vi "Initialize Session without Resources.vi"(11 "error in (no error)":errorcluster) -> (4 "session out":refnum<k21>, 15 "error out":errorcluster)   [LabVIEW 2020, in "SLSC.lvlib"]
doc: "Initializes an SLSC session without specifying any resources or opening any network connections. Use Initialize Session without Resources if you need to set session properties that control network timeouts or the ability to programmatically abort blocking network operations."
uses:
  <vilib>/SLSC/SLSC.lvlib
  nislsclvapi.dll
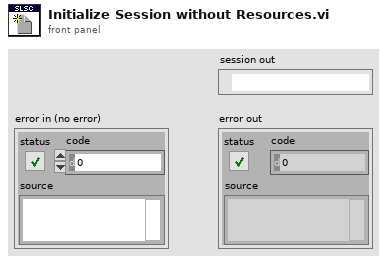
[diagram p1: front panel]
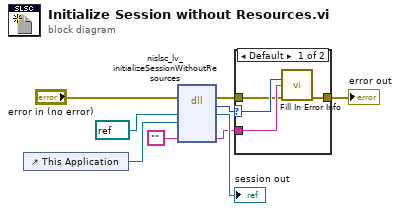
[diagram p0: block diagram]
diagram:
  n1 = control-ref of="This Application"() -> (w1:refnum<vi>)
  n2 = dll-call lib="nislsclvapi.*" fn="nislsc_lv_initializeSessionWithoutResources"(error in="error in (no error)", "session"=refnum<k21> refnum ("SLSC Session"), "lvAppRef"=w1, "extendedErrorInfo"="") -> (error out=w3:errorcluster, "return type"=w5:i32, "session"=→"session out":refnum<k21>, "extendedErrorInfo"=w4:string)  [unwired: 5 in, 1 out]
  n3 = case shown="Default" w5 {
    selector: w5 -> [w13 _]
    tunnel: w4 -> [w12 _]
    tunnel: w3 -> [w11 w14]
    tunnel: [w10 w14] -> w2
    frame Default {
      n4 = call <vilib>:"Fill In Error Info.vi"("status code"=w13, "extended error info"=w12, "error in"=w11) -> ("error out"=w10:errorcluster)  [unwired: 12 in]
    }
    frame 0 {
    }
  }
  "error out" <- w2
